vi "meta_data.vi"(0 "User":string, 5 "Sample Information":string, 9 "SMU1 Terminal":string(combo)) -> (4 "SMU2 Terminal":string, 6 "SMU3 Terminal":string)   [LabVIEW 2021]
panel:
  in  "Estimated Sample Dimensions":string
  out "SMU1 Terminal":string
  in  "SMU3 Description":string
  in  "SMU2 Description":string
  in  "SMU1 Description":string
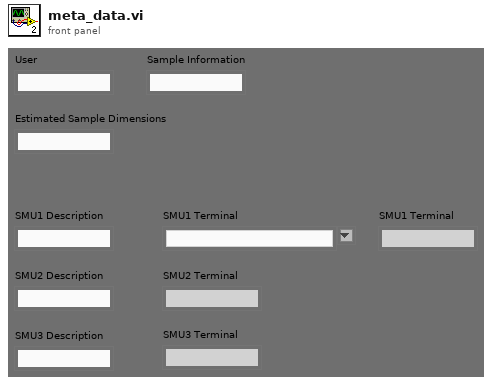
[diagram p1: front panel]
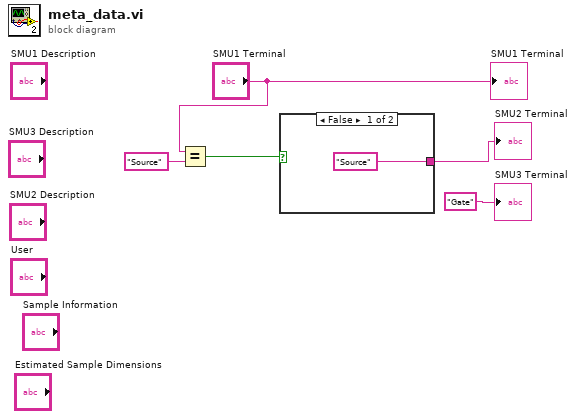
[diagram p0: block diagram]
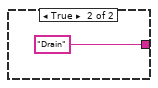
[diagram p2: hidden frame]
diagram:
  n1 = Equal?(x="SMU1 Terminal", y="Source") -> (x = y?=w3:bool)
  n2 = case shown="False" w3 {
    tunnel: ["Source" "Drain"] -> w2
    frame False {
    }
    frame True {
    }
  }
  "SMU2 Terminal" <- w2
  "SMU1 Terminal" <- "SMU1 Terminal"
  "SMU3 Terminal" <- "Gate" ("SMU3 Terminal")
